vi "OLD-Get_4275_Configuration.vi"(8 "error in":errorcluster) -> (0 "error out":errorcluster, 2 "Keystate":string)   [LabVIEW 2020]
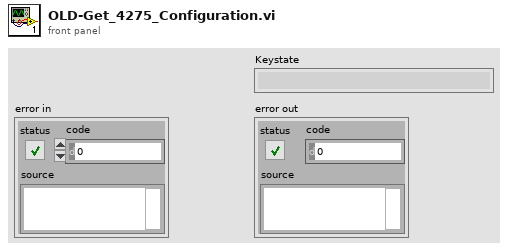
[diagram p1: front panel]
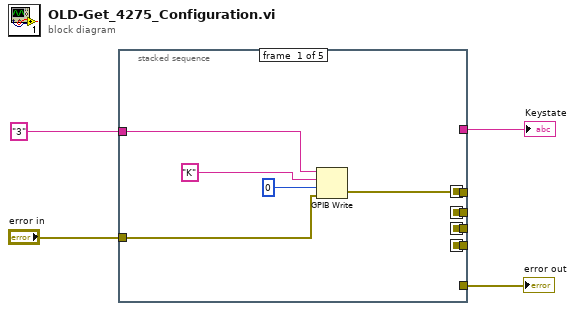
[diagram p0: block diagram]
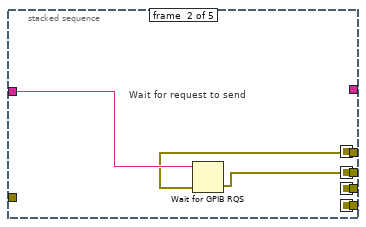
[diagram p2: hidden frame]
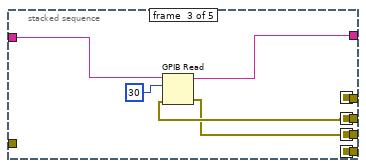
[diagram p3: hidden frame]
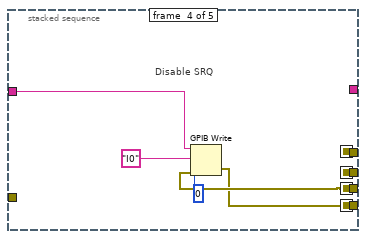
[diagram p4: hidden frame]
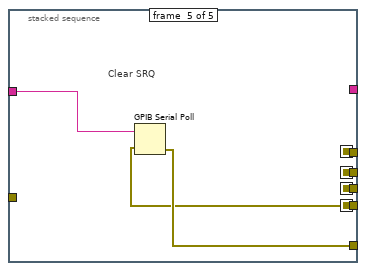
[diagram p5: hidden frame]
diagram:
  n1 = stacked-sequence {
    seq-local: [w5 _ _ _ _] -> [_ w11 _ _ _]
    seq-local: [_ w10 _ _ _] -> [_ _ w14 _ _]
    seq-local: [_ _ w13 _ _] -> [_ _ _ w19 _]
    seq-local: [_ _ _ w18 _] -> [_ _ _ _ w23]
    tunnel: "3" -> [w9 w12 w17 w20 w25]
    tunnel: "error in" -> [w6 _ _ _ _]
    tunnel: [_ _ w15 _ _] -> w3
    tunnel: [_ _ _ _ w24] -> w2
    tunnel: [w5 _ _ _ _] -> _
    tunnel: [_ w10 _ _ _] -> _
    tunnel: [_ _ w13 _ _] -> _
    tunnel: [_ _ _ w18 _] -> _
    frame #0 {
      n2 = GPIB Write(0:w9, 1:"K" ("multi-line string"), 2:i16 0 ("mode (0)"), 3:w6) -> (6:w5:errorcluster)  [unwired: 1 in, 1 out]
    }
    frame #1 {
      # "Wait for request to send"
      n3 = Wait for GPIB RQS(2:w11, 4:w12) -> (0:w10:errorcluster)  [unwired: 1 in, 1 out]
    }
    frame #2 {
      n4 = GPIB Read(0:w17, 1:30 ("byte count"), 3:w14) -> (5:w15:string, 7:w13:errorcluster)  [unwired: 2 in, 1 out]
    }
    frame #3 {
      # "Disable SRQ"
      n5 = GPIB Write(0:w20, 1:"I0", 2:0, 3:w19) -> (6:w18:errorcluster)  [unwired: 1 in, 1 out]
    }
    frame #4 {
      # "Clear SRQ"
      n6 = GPIB Serial Poll(0:w25, 1:w23) -> (4:w24:errorcluster)  [unwired: 2 out]
    }
  }
  "Keystate" <- w3
  "error out" <- w2
